vi "Loop Delay.vi"   [LabVIEW 2014]
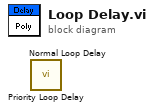
[diagram p0: block diagram]
diagram:
  n1 = call "Priority Loop Delay.vi"() -> ()  [unwired: 11 in, 1 out]
  n2 = call "Normal Loop Delay.vi"() -> ()  [unwired: 11 in, 1 out]
